vi "GA_string_scrub.vi"(8 "error in (no error)":errorcluster, 10 "opMode":enum16{"Warming up", "Runtime"}(ring), 11 "input":string) -> (0 "error out":errorcluster, 1 "Zeroing":bool, 2 "Warming up":bool, 3 "output array":string[](array[string]), 4 "Zeroing count":dbl, 5 "Warm up temp":dbl, 6 "Time":dbl, 7 "output string":string)   [LabVIEW 2016]
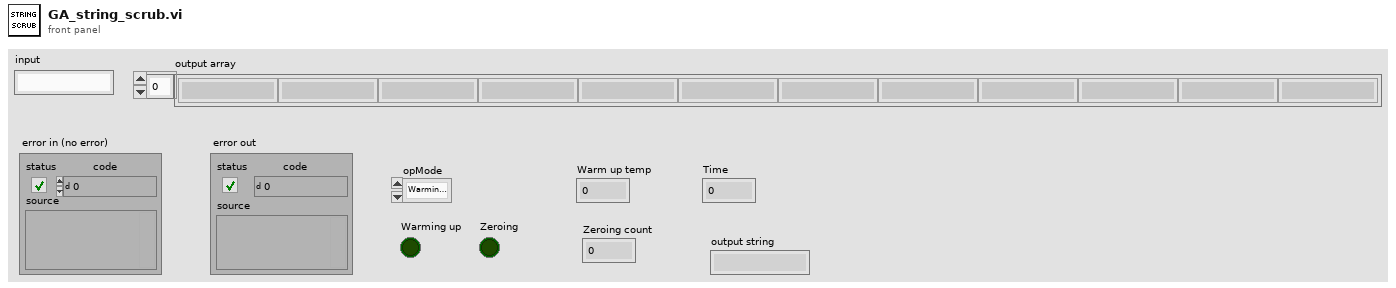
[diagram p1: front panel]
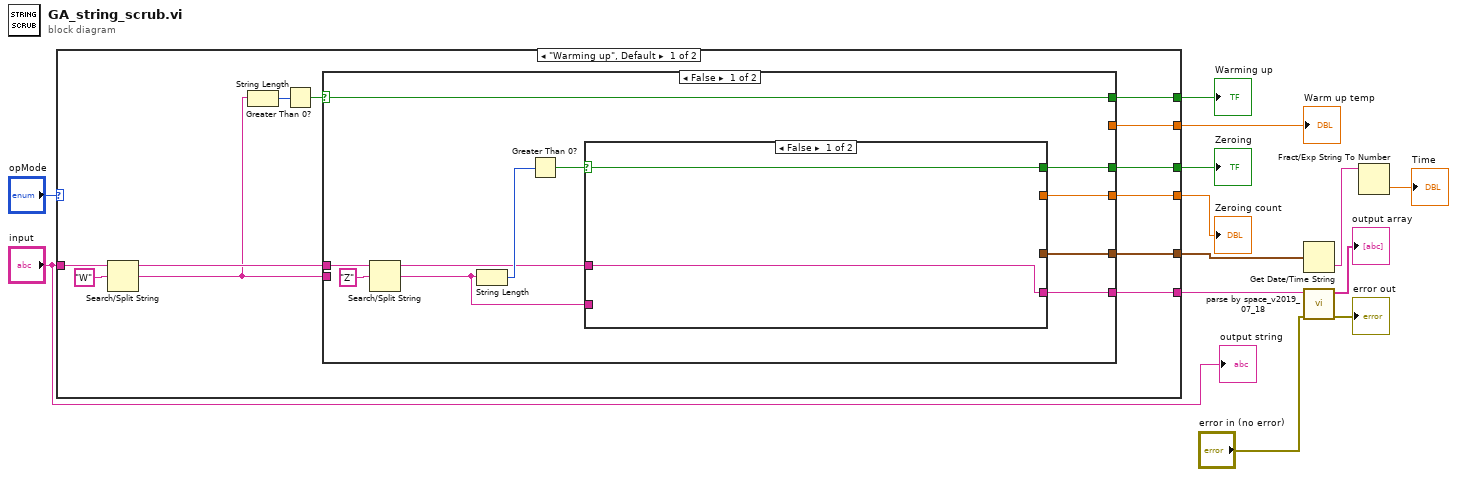
[diagram p0: block diagram]
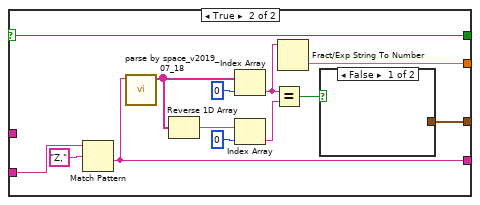
[diagram p2: hidden frame]
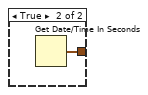
[diagram p3: hidden frame]
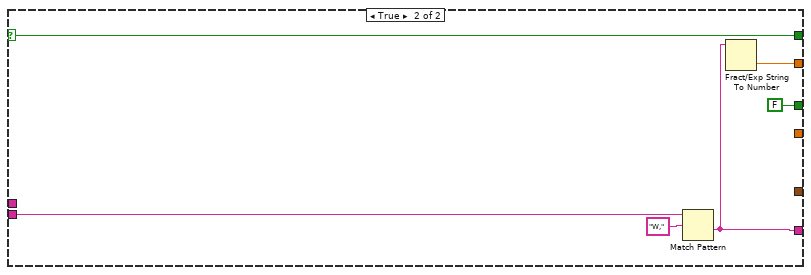
[diagram p4: hidden frame]
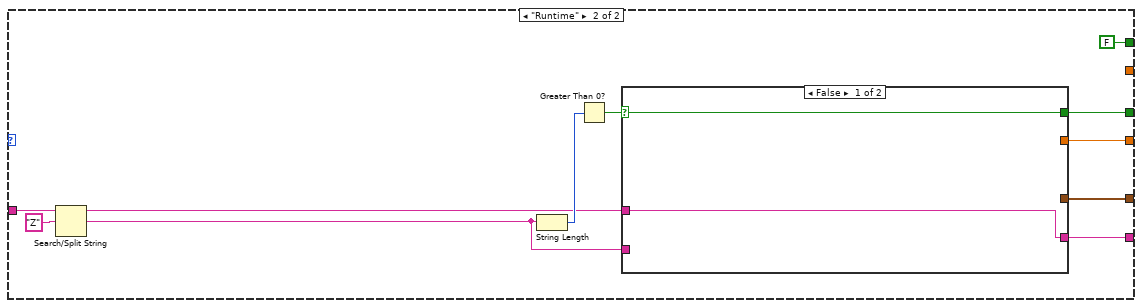
[diagram p5: hidden frame]
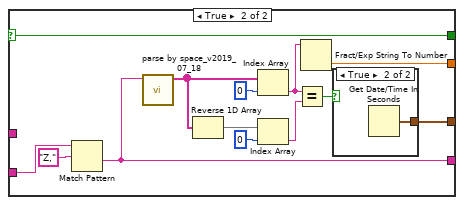
[diagram p6: hidden frame]
diagram:
  n1 = case shown="\"Warming up\", Default" "opMode" {
    tunnel: "input" -> [w25 w64]
    tunnel: [w19 w63] -> w13
    tunnel: [w18 FALSE] -> w8
    tunnel: [w17 w61] -> w7
    tunnel: [w16 _] -> w6
    tunnel: [w15 w60] -> w5
    tunnel: [w14 w59] -> w4
    frame "Warming up", Default {
      n2 = Search/Split String(string=w25, search string/char (-)="W") -> (substring before match=w21:string, match + rest of string=w20:string)  [unwired: 1 in, 1 out]
      n3 = String Length(string=w20) -> (length=w23:i32)
      n4 = Greater Than 0?(x=w23) -> (x > 0?=w22:bool)
      n5 = case shown="False" w22 {
        selector: w22 -> [w29 w56]
        tunnel: w21 -> [w35 _]
        tunnel: w20 -> [_ w58]
        tunnel: [w30 w54] -> w19
        tunnel: [w29 w56] -> w18
        tunnel: [w28 FALSE] -> w17
        tunnel: [_ w53] -> w16
        tunnel: [w27 _] -> w15
        tunnel: [w26 _] -> w14
        frame False {
          n6 = Search/Split String(string=w35, search string/char (-)="Z") -> (substring before match=w31:string, match + rest of string=w32:string)  [unwired: 1 in, 1 out]
          n7 = String Length(string=w32) -> (length=w33:i32)
          n8 = Greater Than 0?(x=w33) -> (x > 0?=w36:bool)
          n9 = case shown="False" w36 {
            selector: w36 -> [w38 w49]
            tunnel: w32 -> [_ w51]
            tunnel: w31 -> [w37 _]
            tunnel: [w37 w48] -> w30
            tunnel: [w38 w49] -> w28
            tunnel: [_ w46] -> w27
            tunnel: [_ w45] -> w26
            frame False {
            }
            frame True {
              n10 = Match Pattern(string=w51, regular expression="Z,") -> (after substring=w48:string)  [unwired: 1 in, 3 out]
              n11 = call "parse by space_v2019_07_18.vi"("String"=w48) -> ("Array"=w42:string[])  [unwired: 9 in, 1 out]
              n12 = Reverse 1D Array(array=w42) -> (reversed array=w41:string[])
              n13 = Index Array(array=w42, index=0) -> (element=w43:string)
              n14 = Index Array(array=w41, index=0) -> (element=w39:string)
              n15 = Equal?(x=w43, y=w39) -> (x = y?=w44:bool)
              n16 = Fract/Exp String To Number(string=w43) -> (number=w46:dbl)  [unwired: 3 in, 1 out]
              n17 = case shown="False" w44 {
                tunnel: [_ w52] -> w45
                frame False {
                }
                frame True {
                  n18 = Get Date/Time In Seconds() -> (seconds since 1Jan1904=w52:timestamp)
                }
              }
            }
          }
        }
        frame True {
          n19 = Match Pattern(string=w58, regular expression="W,") -> (after substring=w54:string)  [unwired: 1 in, 3 out]
          n20 = Fract/Exp String To Number(string=w54) -> (number=w53:dbl)  [unwired: 3 in, 1 out]
        }
      }
    }
    frame "Runtime" {
      n21 = Search/Split String(string=w64, search string/char (-)="Z") -> (substring before match=w65:string, match + rest of string=w66:string)  [unwired: 1 in, 1 out]
      n22 = String Length(string=w66) -> (length=w67:i32)
      n23 = Greater Than 0?(x=w67) -> (x > 0?=w69:bool)
      n24 = case shown="False" w69 {
        selector: w69 -> [w71 w82]
        tunnel: w66 -> [_ w84]
        tunnel: w65 -> [w70 _]
        tunnel: [w70 w81] -> w63
        tunnel: [w71 w82] -> w61
        tunnel: [_ w79] -> w60
        tunnel: [_ w78] -> w59
        frame False {
        }
        frame True {
          n25 = Match Pattern(string=w84, regular expression="Z,") -> (after substring=w81:string)  [unwired: 1 in, 3 out]
          n26 = call "parse by space_v2019_07_18.vi"("String"=w81) -> ("Array"=w75:string[])  [unwired: 9 in, 1 out]
          n27 = Reverse 1D Array(array=w75) -> (reversed array=w74:string[])
          n28 = Index Array(array=w75, index=0) -> (element=w76:string)
          n29 = Index Array(array=w74, index=0) -> (element=w72:string)
          n30 = Equal?(x=w76, y=w72) -> (x = y?=w77:bool)
          n31 = Fract/Exp String To Number(string=w76) -> (number=w79:dbl)  [unwired: 3 in, 1 out]
          n32 = case shown="True" w77 {
            tunnel: [_ w85] -> w78
            frame False {
            }
            frame True {
              n33 = Get Date/Time In Seconds() -> (seconds since 1Jan1904=w85:timestamp)
            }
          }
        }
      }
    }
  }
  "Warming up" <- w8
  "Zeroing" <- w7
  "Warm up temp" <- w6
  "Zeroing count" <- w5
  n34 = Get Date/Time String(seconds (now)=w4) -> (time string=w3:string)  [unwired: 2 in, 1 out]
  n35 = call "parse by space_v2019_07_18.vi"("error in (no error)"="error in (no error)", "String"=w13) -> ("error out"=→"error out":errorcluster, "Array"=→"output array":string[])  [unwired: 8 in]
  n36 = Fract/Exp String To Number(string=w3) -> (number=→"Time":dbl)  [unwired: 3 in, 1 out]
  "output string" <- "input"
